vi "Attach Bus Monitor.vi"(10 "BusMonitor":refnum<class "IBusMonitor.lvclass">, 11 "MonitoredMediator in":refnum<class "MonitoredMediator.lvclass">) -> (3 "MonitoredMediator out":refnum<class "MonitoredMediator.lvclass">)   [LabVIEW 2018, in "MVA Framework.lvlib" / "MonitoredMediator.lvlib" / "MonitoredMediator.lvclass"]
doc: "附加总线监视器"
uses:
  MonitoredMediator.lvclass
  Mediator/Mediator/Mediator.lvclass
  Mediator/Topic Messages/Add Topic Subscriber Msg/Add Topic Subscriber Msg.lvclass
  Mediator/TopicLookupTable/TopicLookupTable.lvclass
  IMediator/ISubscriptionPolicy/ISubscriptionPolicy.lvclass
  IBusMonitor/IBusMonitor.lvclass
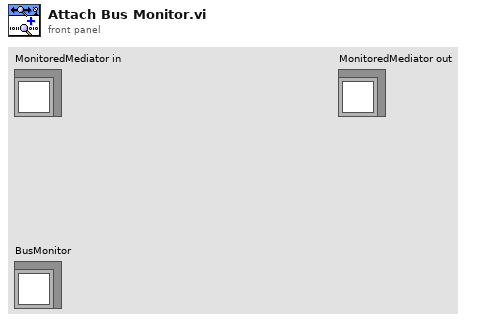
[diagram p1: front panel]
types:
  T1 = typedef "MVA Framework.lvlib/IMediator.lvlib/ISubscriptionPolicy.lvclass/ISubscriptionPolicy Reference.ctl" = refnum<data-value>
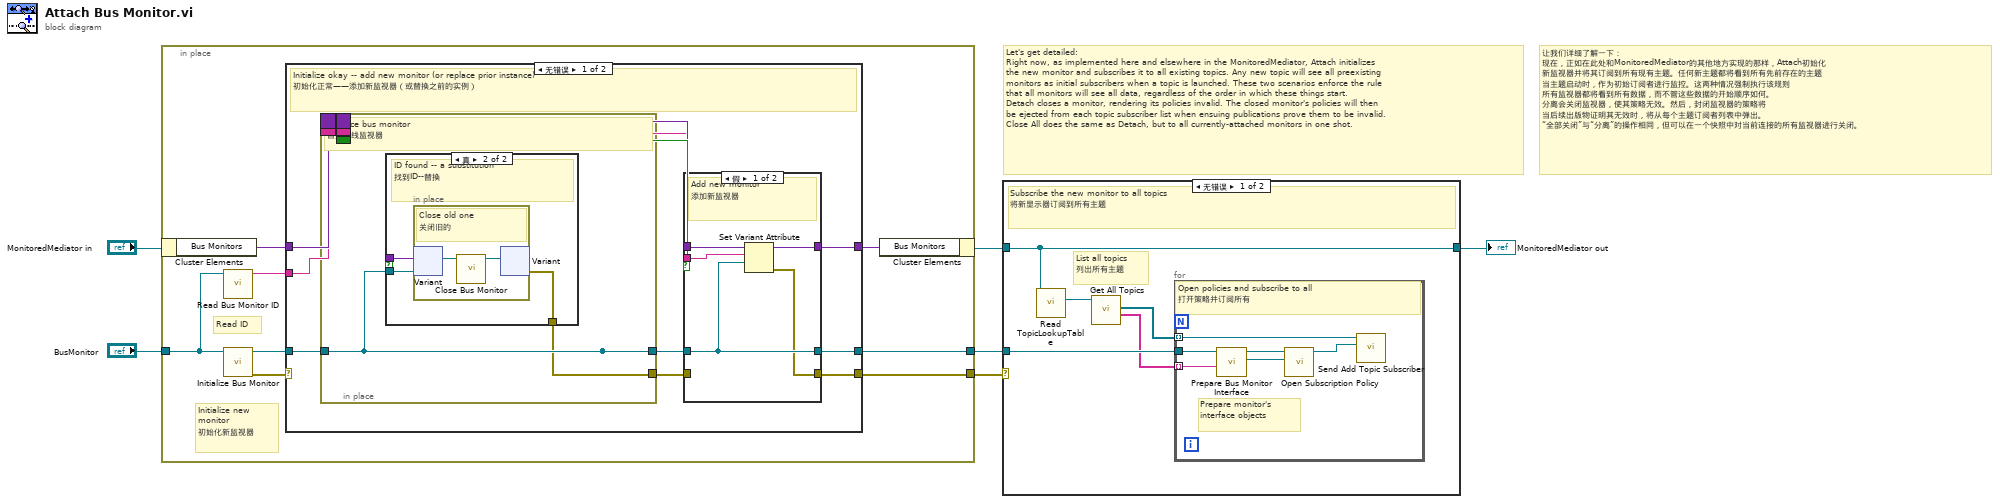
[diagram p0: block diagram]
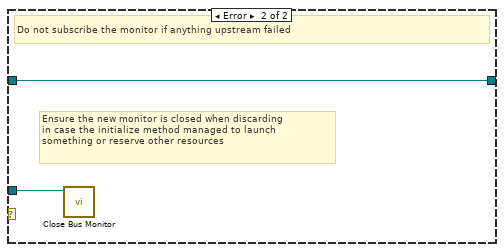
[diagram p5: hidden frame]
diagram:
  # "让我们详细了解一下：\n现在，正如在此处和MonitoredMediator的其他地方实现的那样，Attach初始化\n新监视器并将其订阅到所有现有主题。任何新主题都将看到所有先前存在的主题\n当主题启动时，作为初始订阅者进行监控。这两种情况强制执行该规则\n所有监视器都将看到所有数据，而不管这些数据的开始顺序如何。\n分离会关闭监视器，使其策略无效。然后，封闭监视器的策略将\n当后续出版物证明其无效时，将从每个主题订阅者列表中弹出。\n“全部关闭”与“分离”的操作相同，但可以在一个快照中对当前连接的所有监视器进行关闭。"
  # "Let's get detailed:\nRight now, as implemented here and elsewhere in the MonitoredMediator, Attach initializes\nthe new monitor and subscribes it to all existing topics. Any new topic will see all preexisting\nmonitors as initial subscribers when a topic is launched. These two scenarios enforce the rule\nthat all monitors will see all data, regardless of the order in which these things start.\nDetach closes a monitor, rendering its policies invalid. The closed monitor's policies will then\nbe ejected from each topic subscriber list when ensuing publications prove them to be invalid.\nClose All does the same as Detach, but to all currently-attached monitors in one shot."
  n1 = in-place {
    in-place-border: "BusMonitor" -> [w8]
    in-place-border: [w10] -> w3
    in-place-border: [w7] -> w1
    # "Read ID"
    # "Initialize new\nmonitor\n初始化新监视器"
    n2 = in-place-cluster #1("MonitoredMediator in") -> ("Bus Monitors"=w13:variant)
    n3 = call-dynamic "Read Bus Monitor ID.vi"("IBusMonitor"=w8) -> ("Bus Monitor ID"=w9:string)  [unwired: 10 in]
    n4 = call-dynamic "Initialize Bus Monitor.vi"("IBusMonitor In"=w8) -> ("error out"=w14:errorcluster, "IBusMonitor Out"=w12:refnum<class "IBusMonitor.lvclass">)  [unwired: 9 in]
    n5 = case shown="无错误" w14 {
      selector: w14 -> [_ w44]
      tunnel: w13 -> [w25 w45]
      tunnel: w12 -> [w24 w43]
      tunnel: [w19 w45] -> w11
      tunnel: [w18 w44] -> w10
      tunnel: w9 -> [w16 _]
      tunnel: [w15 w43] -> w7
      frame No Error {
        # "Initialize okay -- add new monitor (or replace prior instance)\n初始化正常——添加新监视器（或替换之前的实例）"
        n6 = in-place {
          border: w25 -> [_]
          border: w16 -> [_]
          border: [_] -> w22
          border: [_] -> w21
          border: [_] -> w23
          in-place-border: w24 -> [w35]
          in-place-border: [w35] -> w20
          in-place-border: [w34] -> w17
          # "Replace bus monitor\n替换总线监视器"
          n7 = case shown="真" w36 {
            tunnel: w37 -> [_ w40]
            tunnel: w35 -> [_ w39]
            tunnel: [_ w38] -> w34
            frame False {
              # "Nothing to close"
              # "Old ID not found"
            }
            frame True {
              # "ID found -- a substitution\n找到ID--替换"
              n8 = in-place {
                # "Close old one\n关闭旧的"
                n9 = in-place-variant #2(w40, w39) -> (w42:refnum<class "IBusMonitor.lvclass">)  [unwired: 1 out]
                n10 = call-dynamic "Close Bus Monitor.vi"("IBusMonitor In"=w42) -> ("IBusMonitor Out"=w41:refnum<class "IBusMonitor.lvclass">)  [unwired: 10 in]
                n11 = in-place-variant #2(w41) -> (w38:errorcluster)  [unwired: 1 out]
              }
            }
          }
        }
        n12 = case shown="假" w23 {
          tunnel: w22 -> [w30 w33]
          tunnel: w21 -> [w29 _]
          tunnel: w20 -> [w27 w31]
          tunnel: [w28 w33] -> w19
          tunnel: [w26 w32] -> w18
          tunnel: w17 -> [_ w32]
          tunnel: [w27 w31] -> w15
          frame False {
            # "Add new monitor\n添加新监视器"
            n13 = Set Variant Attribute(Variant=w30, name=w29, value=w27) -> (Variant out=w28:variant, error out=w26:errorcluster)  [unwired: 1 in, 1 out]
          }
          frame True {
            # "This was a substitution"
          }
        }
      }
      frame Error {
        # "Do not add new monitor if initialization fails"
      }
    }
    n14 = in-place-cluster #1("Bus Monitors"=w11) -> (w4:refnum<class "MonitoredMediator.lvclass">)
  }
  n15 = case shown="无错误" w3 {
    tunnel: w4 -> [w48 w58]
    tunnel: [w48 w58] -> w2
    tunnel: w1 -> [w47 w57]
    frame No Error {
      # "List all topics\n列出所有主题"
      # "Subscribe the new monitor to all topics\n将新显示器订阅到所有主题"
      n16 = call "Read TopicLookupTable.vi"("Mediator in"=w48) -> ("TopicLookupTable"=w50:refnum<data-value>)  [unwired: 10 in]
      n17 = call "Get All Topics.vi"("TopicLookupTable"=w50) -> ("Topic Names"=w46:string[], "Topic Enqueuers"=w49:refnum<class "Message Enqueuer.lvclass">[])  [unwired: 7 in, 2 out]
      n18 = for {
        tunnel: w49 -> [w56] mode=indexing
        tunnel: w46 -> [w53] mode=indexing
        tunnel: w47 -> [w54]
        # "Prepare monitor's\ninterface objects"
        # "Open policies and subscribe to all\n打开策略并订阅所有"
        n19 = call-dynamic "Prepare Bus Monitor Interface.vi"("Datum Name"=w53, "IBusMonitor"=w54) -> ("Valid Transport"=w51:refnum<class "ITransport.lvclass">, "SubscriptionPolicy"=w52:refnum<class "ISubscriptionPolicy.lvclass">)  [unwired: 8 in]
        n20 = call "Open Subscription Policy.vi"("Transport"=w51, "SubscriptionPolicy"=w52) -> ("Subscription Policy"=w55:T1)  [unwired: 8 in, 1 out]
        n21 = call "Send Add Topic Subscriber.vi"("Subscription Policy"=w55, "Message Enqueuer"=w56) -> ()  [unwired: 8 in, 2 out]
      }
    }
    frame Error {
      # "Ensure the new monitor is closed when discarding\nin case the initialize method managed to launch\nsomething or reserve other resources"
      # "Do not subscribe the monitor if anything upstream failed"
      n22 = call-dynamic "Close Bus Monitor.vi"("IBusMonitor In"=w57) -> ()  [unwired: 10 in, 1 out]
    }
  }
  "MonitoredMediator out" <- w2
